vi "Main.vi"(11 "Module Admin":refnum<class "Delacor_lib_QMH_Module Admin.lvclass">) -> ()   [LabVIEW 2025, in "Number Pad.lvlib"]
doc: "This template is based off of the Queued Message Handler design pattern and the Queued Message Handler project template that ships with LabVIEW.\n\nThe main difference is that the queue is private to this module and communication between modules is performed via Broadcast and Request events.\n\nRequest events are wrapped in public API methods and are handled in the Event Handling Loop (EHL) of this VI. Any module can register for Broadcast events sent by this module. The EHL generates messages based on user interface actions.\n\nThe Message Handling Loop (MHL) processes messages generated by the EHL, or by other messages. The messages are string values, so new messages can be added easily to the Message Cases case structure in the MHL. Each message cluster can also provide an optional value for Message Data, which is a variant that can be converted to whatever message-specific data is required.\n_____\nBased on DQMH Dev Tools: Project Template 7.1.0.1503."
uses:
  Number Pad.lvlib
  <vilib>/Delacor/Delacor QMH/Libraries/Module Admin_class/Delacor_lib_QMH_Module Admin.lvclass
  Module Data--cluster.ctl
  <vilib>/Delacor/Delacor QMH/Libraries/Message Queue_class/Delacor_lib_QMH_Message Queue.lvclass/Delacor_lib_QMH_Message Queue.ctl
  Stop Argument--cluster.ctl
  <vilib>/Delacor/Delacor QMH/Libraries/Module Admin_class/Delacor_lib_QMH_Module Admin.lvclass/Delacor_lib_QMH_Module Admin.ctl
  Get VI refnum Argument--cluster.ctl
  Get VI refnum (Reply Payload)--cluster.ctl
  <vilib>/Utility/miscctls.llb/LVPointTypeDef.ctl
  <vilib>/Delacor/Delacor QMH/Libraries/Message Queue_class/Delacor_lib_QMH_Enqueue Message (Single).vi
  <vilib>/Delacor/Delacor QMH/Libraries/Module Admin_class/Delacor_lib_QMH_Get External Launch.vi
  <vilib>/Delacor/Delacor QMH/Libraries/Message Queue_class/Delacor_lib_QMH_Message Queue.lvclass
panel:
  in  "Enter":bool
  out "Buffer Indicator":string
  in  "CLR":bool
  in  "BS":bool
  in  ".":bool
  in  "0":bool
  in  "9":bool
  in  "8":bool
  in  "7":bool
  in  "6":bool
  in  "5":bool
  in  "4":bool
  in  "3":bool
  in  "2":bool
  in  "1":bool
  out "error out":errorcluster
  out "Status":string
  in  "Simulate MHL Error":bool
  in  "Simulate EHL Error":bool
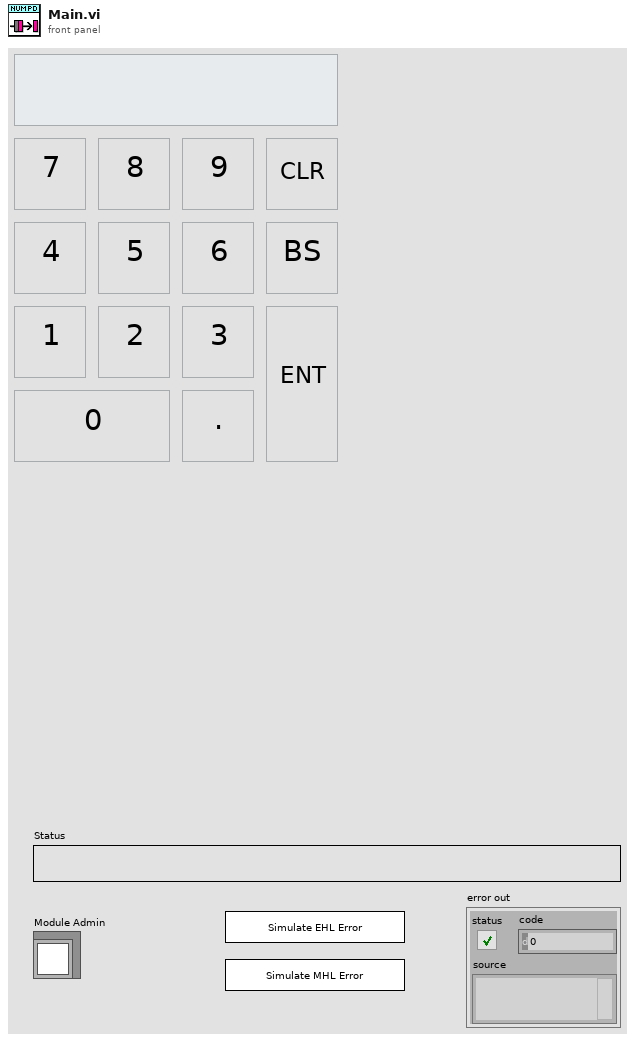
[diagram p1: front panel]
types:
  T1 = typedef "Number Pad.lvlib/Request Events--cluster.ctl" = cluster{"Stop Module":refnum<user-event>, "Show Panel":refnum<user-event>, "Hide Panel":refnum<user-event>, "Get Module Execution Status":refnum<user-event>, "Show Diagram":refnum<user-event>, "Get VI refnum":refnum<user-event>}
  T2 = typedef "Number Pad.lvlib/Module Data--cluster.ctl" = cluster{"Status":string, "Buffer":string}
  T3 = enum32{"invalid lock state", "Not Locked", "Locked (No Password)", "Password-protected"}
  T4 = typedef "Number Pad.lvlib/Stop Argument--cluster.ctl" = cluster{"Origin":string, "Exit via Stop Module Req?":bool, "Wait for Module to stop?":bool}
  T5 = typedef "Number Pad.lvlib/Get VI refnum Argument--cluster.ctl" = cluster{"Wait Notifier":refnum<notifier>, "wait for reply":bool}
  T6 = typedef "LVPointTypeDef.ctl" = cluster{"Horizontal":i16, "Vertical":i16}
  T7 = enum32{"Invalid", "Standard", "Closed", "Hidden", "Minimized", "Maximized"}
  T8 = typedef "Number Pad.lvlib/Get VI refnum (Reply Payload)--cluster.ctl" = cluster{"VI Refnum":refnum<vi>, "error":errorcluster}
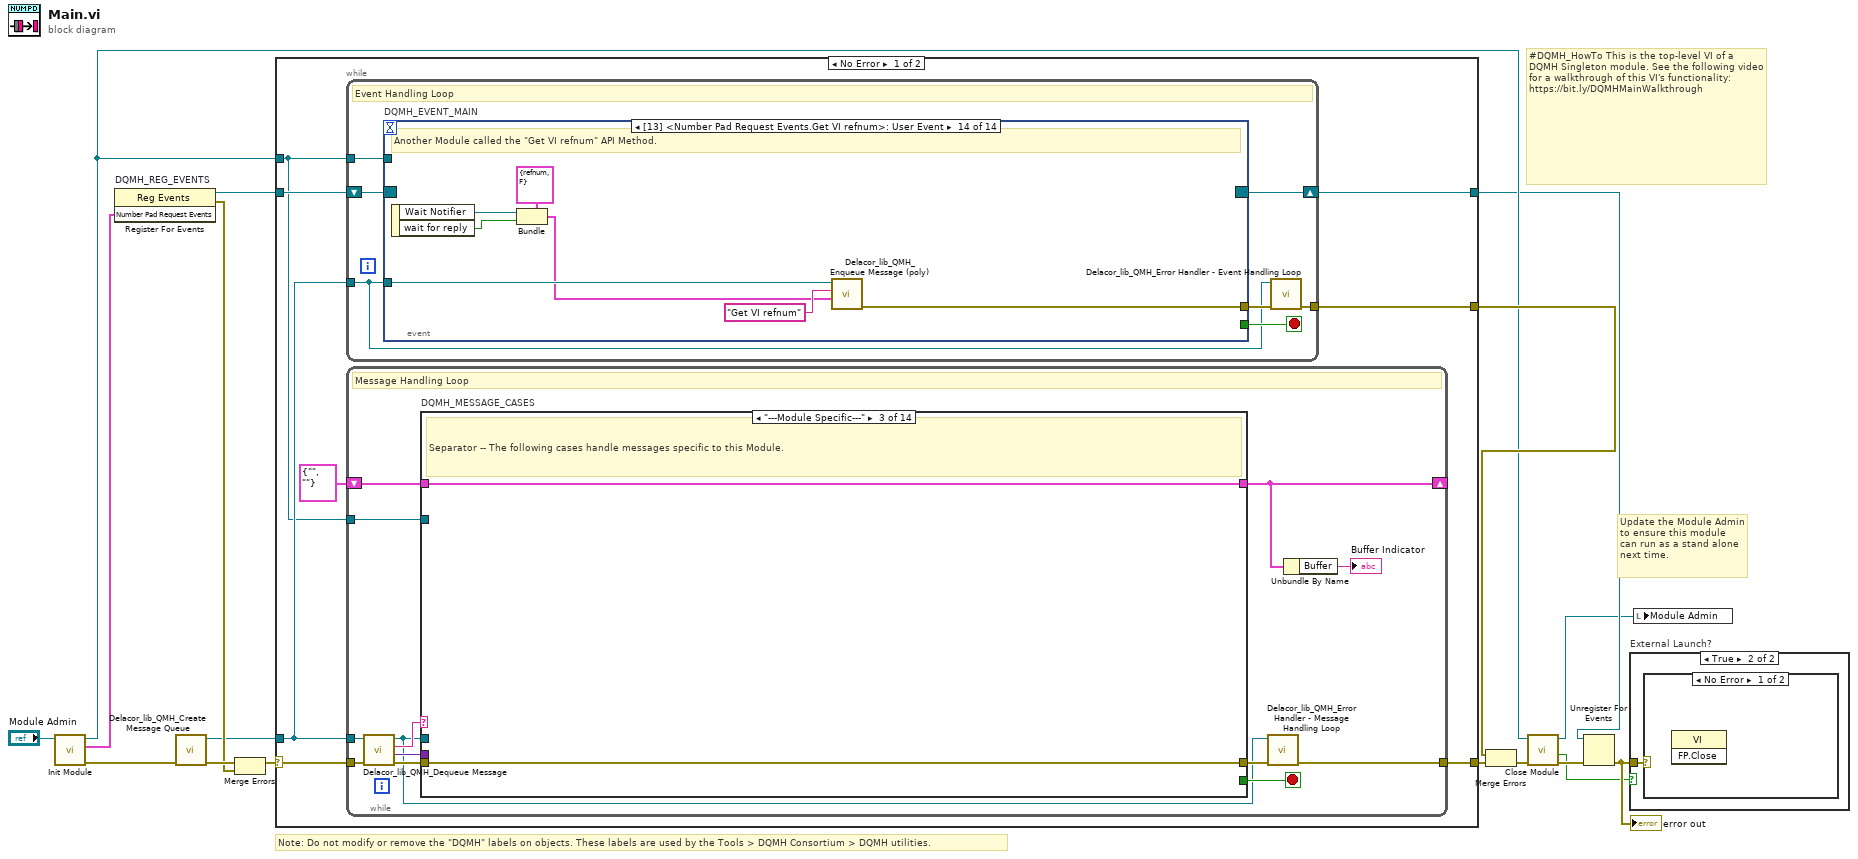
[diagram p0: block diagram]
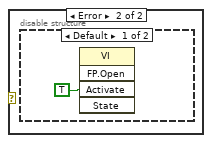
[diagram p3: hidden frame]
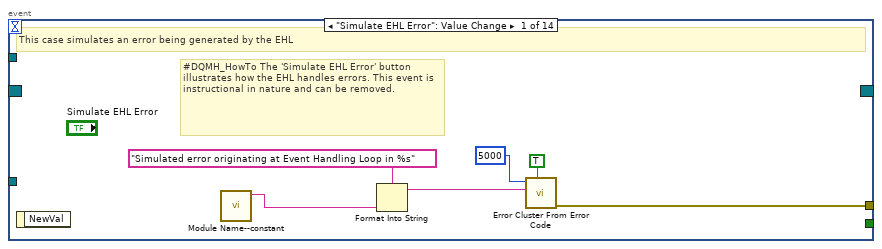
[diagram p5: hidden frame]
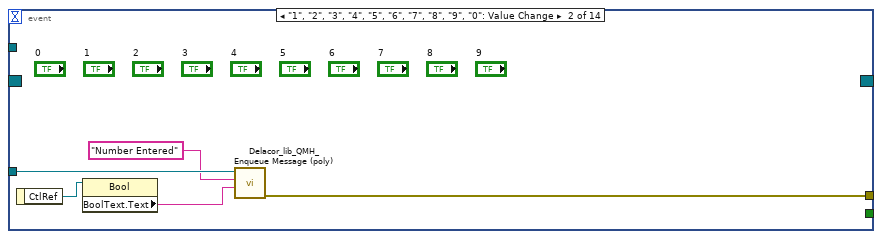
[diagram p6: hidden frame]
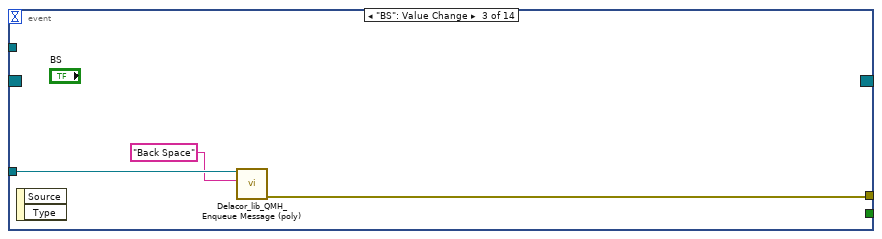
[diagram p7: hidden frame]
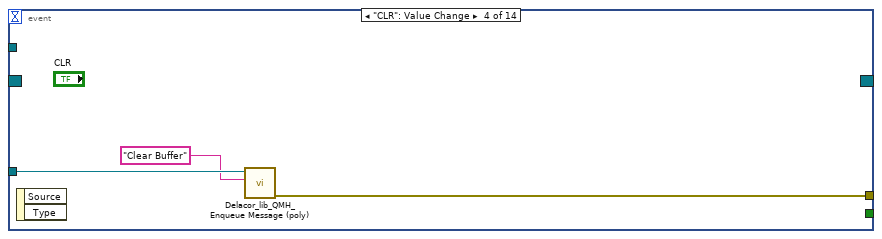
[diagram p8: hidden frame]
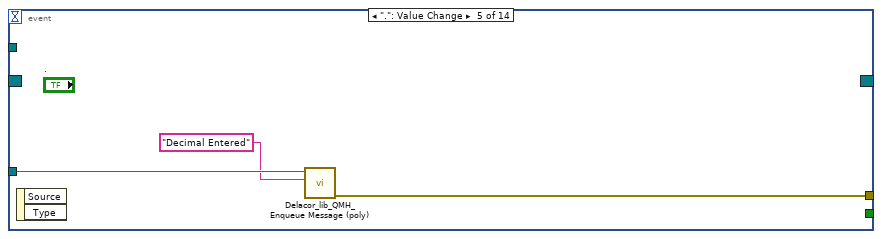
[diagram p9: hidden frame]
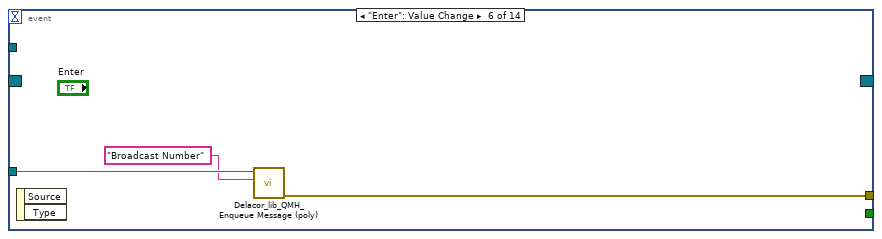
[diagram p10: hidden frame]
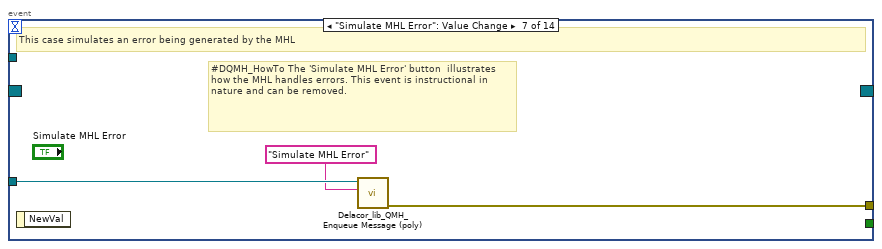
[diagram p11: hidden frame]
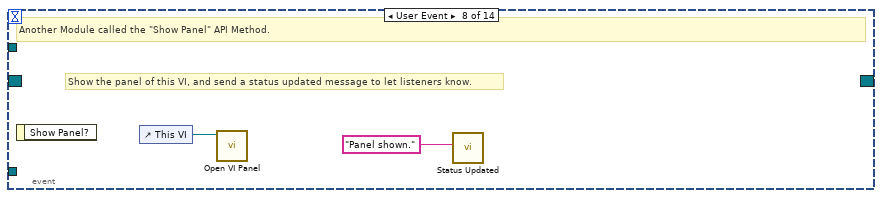
[diagram p12: hidden frame]
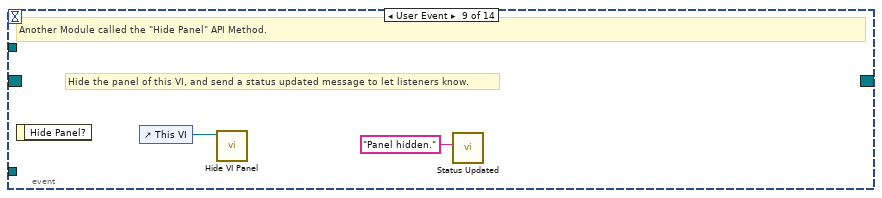
[diagram p13: hidden frame]
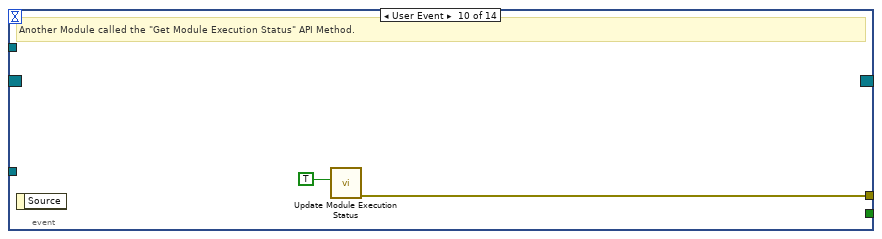
[diagram p14: hidden frame]
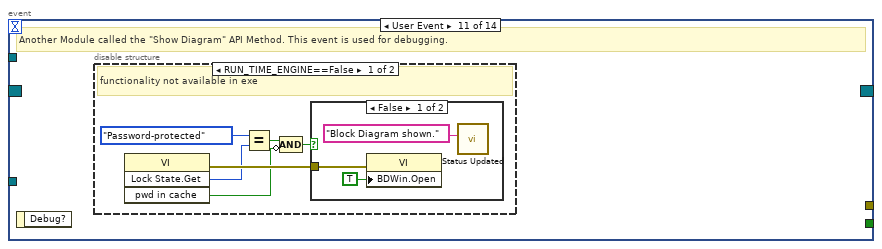
[diagram p15: hidden frame]
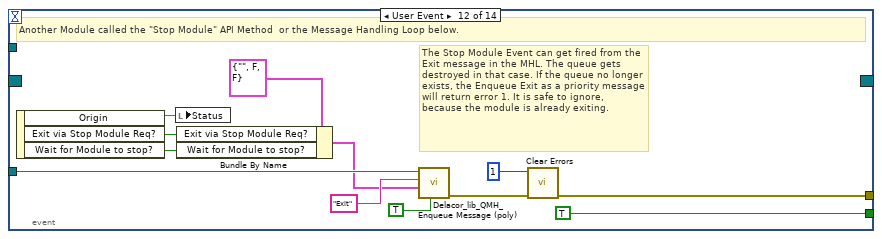
[diagram p18: hidden frame]
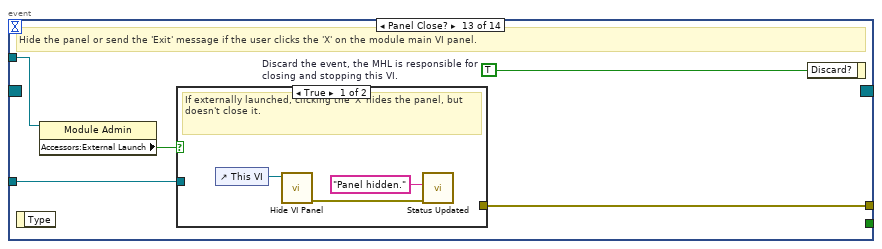
[diagram p19: hidden frame]
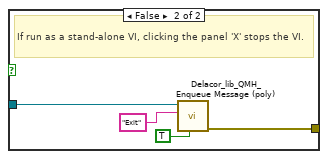
[diagram p20: hidden frame]
diagram:
  # "#DQMH_HowTo This is the top-level VI of a DQMH Singleton module. See the following video for a walkthrough of this VI's functionality: https://bit.ly/DQMHMainWalkthrough"
  # "Note: Do not modify or remove the \"DQMH\" labels on objects. These labels are used by the Tools > DQMH Consortium > DQMH utilities."
  # "Update the Module Admin to ensure this module can run as a stand alone next time."
  n1 = call "Init Module.vi"("Singleton Module Admin in"="Module Admin") -> ("error out"=w16:errorcluster, "Number Pad Request Events"=w5:T1, "Singleton Module Admin out"=w8:refnum<class "Delacor_lib_QMH_Module Admin.lvclass">)  [unwired: 8 in]
  n2 = register-events "DQMH_REG_EVENTS"(w5) -> (reference out=w6:refnum<event-registration>, error out=w9:errorcluster)  [unwired: 2 in]
  n3 = call <vilib>:"Delacor_lib_QMH_Create Message Queue.vi"("error in"=w16) -> ("error out"=w11:errorcluster, "Message Queue"=w4:refnum<class "Delacor_lib_QMH_Message Queue.lvclass">)  [unwired: 9 in]
  n4 = Merge Errors(w11, w9) -> (w10:errorcluster)
  n5 = case shown="No Error" w10 {
    selector: w10 -> [w23 w265]
    tunnel: [w25 w264] -> w17
    tunnel: [w22 w263] -> w7
    tunnel: w6 -> [w20 w263]
    tunnel: w4 -> [w19 w258]
    tunnel: [w24 _] -> w14
    tunnel: w8 -> [w18 w259]
    frame No Error {
      n6 = while {
        tunnel: w19 -> [w26]
        shift-right: [w29] -> w22
        shift-left: w20 -> [w30]
        tunnel: [w31] -> w24
        tunnel: w18 -> [w27]
        stop <- w28 stop-if-true
        # "Event Handling Loop"
        n7 = event "DQMH_EVENT_MAIN" shown="[13] <Number Pad Request Events.Get VI refnum>: User Event" {
          selector: w30 -> [_ _ _ _ _ _ _ _ _ _ _ _ _ _]
          dyn-events: [_ _ _ _ _ _ _ _ _ _ _ _ _ _] -> w29
          timeout: _ -> [_ _ _ _ _ _ _ _ _ _ _ _ _ _]
          tunnel: [_ _ _ _ _ _ _ _ _ _ _ TRUE ("Discard?") _ _] -> w28
          tunnel: w26 -> [_ w43 w46 w49 w52 w55 w57 _ _ _ _ w81 w88 w104]
          tunnel: [w38 w42 w45 w48 w51 w54 w58 _ _ w64 _ w84 w90 w98] -> w32
          tunnel: w27 -> [_ _ _ _ _ _ _ _ _ _ _ _ w87 _]
          event "Simulate EHL Error": Value Change {
            # "#DQMH_HowTo The 'Simulate EHL Error' button  illustrates how the EHL handles errors. This event is instructional in nature and can be removed."
            # "This case simulates an error being generated by the EHL"
            n8 = event-data() -> ()  [unwired: 1 in, 1 out]
            n9 = call "Module Name--constant.vi"() -> ("Module Name"=w35:string)  [unwired: 11 in]
            n10 = Format Into String(format string="Simulated error originating at Event Handling Loop in %s", w35) -> (resulting string=w36:string)  [unwired: 2 in, 1 out]
            n11 = call <vilib>:"Error Cluster From Error Code.vi"("show call chain? (False)"=TRUE, "error message (\"\")"=w36, "error code (0)"=5000) -> ("error out"=w38:errorcluster)  [unwired: 6 in]
          }
          event "1", "2", "3", "4", "5", "6", "7", "8", "9", "0": Value Change {
            n12 = event-data() -> ("CtlRef"=w40:refnum<vi>)  [unwired: 1 in]
            n13 = property class="Bool"(reference=w40) -> ("BoolText.Text"=w39:string)  [unwired: 1 in, 2 out]
            n14 = call-poly <vilib>:"Delacor_lib_QMH_Enqueue Message (poly).vi"("Message Data"=w39, "Message"="Number Entered", "Message Queue in"=w43) -> ("error out"=w42:errorcluster)  [unwired: 7 in, 1 out]
          }
          event "BS": Value Change {
            n15 = event-data() -> ()  [unwired: 1 in, 2 out]
            n16 = call-poly <vilib>:"Delacor_lib_QMH_Enqueue Message (poly).vi"("Message"="Back Space", "Message Queue in"=w46) -> ("error out"=w45:errorcluster)  [unwired: 8 in, 1 out]
          }
          event "CLR": Value Change {
            n17 = event-data() -> ()  [unwired: 1 in, 2 out]
            n18 = call-poly <vilib>:"Delacor_lib_QMH_Enqueue Message (poly).vi"("Message"="Clear Buffer", "Message Queue in"=w49) -> ("error out"=w48:errorcluster)  [unwired: 8 in, 1 out]
          }
          event ".": Value Change {
            n19 = event-data() -> ()  [unwired: 1 in, 2 out]
            n20 = call-poly <vilib>:"Delacor_lib_QMH_Enqueue Message (poly).vi"("Message"="Decimal Entered", "Message Queue in"=w52) -> ("error out"=w51:errorcluster)  [unwired: 8 in, 1 out]
          }
          event "Enter": Value Change {
            n21 = event-data() -> ()  [unwired: 1 in, 2 out]
            n22 = call-poly <vilib>:"Delacor_lib_QMH_Enqueue Message (poly).vi"("Message"="Broadcast Number", "Message Queue in"=w55) -> ("error out"=w54:errorcluster)  [unwired: 8 in, 1 out]
          }
          event "Simulate MHL Error": Value Change {
            # "#DQMH_HowTo The 'Simulate MHL Error' button  illustrates how the MHL handles errors. This event is instructional in nature and can be removed."
            # "This case simulates an error being generated by the MHL"
            n23 = event-data() -> ()  [unwired: 1 in, 1 out]
            n24 = call-poly <vilib>:"Delacor_lib_QMH_Enqueue Message (poly).vi"("Message"="Simulate MHL Error", "Message Queue in"=w57) -> ("error out"=w58:errorcluster)  [unwired: 8 in, 1 out]
          }
          event User Event {
            # "Show the panel of this VI, and send a status updated message to let listeners know."
            # "Another Module called the \"Show Panel\" API Method."
            n25 = event-data() -> ()  [unwired: 1 in, 1 out]
            n26 = control-ref of="This VI"() -> (w60:refnum<vi>)
            n27 = call "Open VI Panel.vi"("VI"=w60) -> ()  [unwired: 10 in, 1 out]
            n28 = call "Status Updated.vi"("Status"="Panel shown." ("format string")) -> ()  [unwired: 10 in, 1 out]
          }
          event User Event {
            # "Hide the panel of this VI, and send a status updated message to let listeners know."
            # "Another Module called the \"Hide Panel\" API Method."
            n29 = event-data() -> ()  [unwired: 1 in, 1 out]
            n30 = control-ref of="This VI"() -> (w62:refnum<vi>)
            n31 = call "Hide VI Panel.vi"("VI"=w62) -> ()  [unwired: 10 in, 1 out]
            n32 = call "Status Updated.vi"("Status"="Panel hidden." ("format string")) -> ()  [unwired: 10 in, 1 out]
          }
          event User Event {
            # "Another Module called the \"Get Module Execution Status\" API Method."
            n33 = event-data() -> ()  [unwired: 1 in, 1 out]
            n34 = call "Update Module Execution Status.vi"("Running?"=TRUE) -> ("error out"=w64:errorcluster)  [unwired: 10 in]
          }
          event User Event {
            # "Another Module called the \"Show Diagram\" API Method. This event is used for debugging."
            n35 = event-data() -> ()  [unwired: 1 in, 1 out]
            n36 = disable-structure shown="RUN_TIME_ENGINE==False" {
              frame condition #0 (active) {
                # "functionality not available in exe"
                n37 = invoke on="Invoke Node" class="VI" method="Lock State.Get"() -> (error out=w70:errorcluster, "Get Lock State"=w69:T3, "pwd in cache"=w66:bool)  [unwired: 4 in, 1 out]
                n38 = Equal?(x=T3."Password-protected", y=w69) -> (x = y?=w67:bool)
                n39 = Compound Arithmetic op=AND(w67, invert w66) -> (w65:bool)
                n40 = case shown="False" w65 {
                  tunnel: w70 -> [w73 _]
                  frame False {
                    n41 = property on="Property Node" class="VI"(error in=w73, "BDWin.Open"=TRUE ("Block Diagram Window:Open")) -> ()  [unwired: 1 in, 2 out]
                    n42 = call "Status Updated.vi"("Status"="Block Diagram shown." ("format string")) -> ()  [unwired: 10 in, 1 out]
                  }
                  frame True {
                    # "Password-protected VI, and the password is not in the cache. Do not show the diagram."
                  }
                }
              }
              frame condition #1 {
              }
            }
          }
          event User Event {
            # "The Stop Module Event can get fired from the Exit message in the MHL. The queue gets destroyed in that case. If the queue no longer exists, the Enqueue Exit as a priority message will return error 1. It is safe to ignore, because the module is already exiting."
            # "Another Module called the \"Stop Module\" API Method  or the Message Handling Loop below."
            n43 = event-data() -> ("Origin"=w80:string, "Exit via Stop Module Req?"=w76:bool, "Wait for Module to stop?"=w75:bool)  [unwired: 1 in]
            n44 = local write "Status"(w80) -> ()
            n45 = Bundle By Name(cluster=T4 {"Origin"="", "Exit via Stop Module Req?"=FALSE, "Wait for Module to stop?"=FALSE} ("Stop Argument"), "Exit via Stop Module Req?"=w76, "Wait for Module to stop?"=w75) -> (w74:T4)
            n46 = call-poly <vilib>:"Delacor_lib_QMH_Enqueue Message (poly).vi"("Priority Message? (F)"=TRUE, "Message Data"=w74, "Message"="Exit", "Message Queue in"=w81) -> ("error out"=w85:errorcluster)  [unwired: 6 in, 1 out]
            n47 = call <vilib>:"Clear Errors.vi"("error in (no error)"=w85, "specific error code to clear (0: all)"=1) -> ("error out"=w84:errorcluster)  [unwired: 4 in, 1 out]
          }
          event Panel Close? {
            w89 = TRUE  # Discard the event, the MHL is responsible for closing and stopping this VI.
            # "Hide the panel or send the 'Exit' message if the user clicks the 'X' on the module main VI panel."
            n48 = event-data() -> ()  [unwired: 1 in, 1 out]
            n49 = property on="Property Node" class="Module Admin"(reference=w87) -> ("Accessors:External Launch"=w86:bool)  [unwired: 1 in, 2 out]
            n50 = case shown="True" w86 {
              tunnel: w88 -> [_ w96]
              tunnel: [_ w97] -> w90
              frame True {
                # "If externally launched, clicking the 'X' hides the panel, but doesn't close it."
                n51 = control-ref of="This VI"() -> (w93:refnum<vi>)
                n52 = call "Hide VI Panel.vi"("VI"=w93) -> ("error out"=w91:errorcluster)  [unwired: 10 in]
                n53 = call "Status Updated.vi"("error in"=w91, "Status"="Panel hidden." ("format string")) -> ()  [unwired: 9 in, 1 out]
              }
              frame False {
                # "If run as a stand-alone VI, clicking the panel 'X' stops the VI."
                n54 = call-poly <vilib>:"Delacor_lib_QMH_Enqueue Message (poly).vi"("Priority Message? (F)"=TRUE, "Message"="Exit", "Message Queue in"=w96) -> ("error out"=w97:errorcluster)  [unwired: 7 in, 1 out]
              }
            }
            n55 = event-data ("Event Filter Node")("Discard?"=w89) -> ()  [unwired: 1 in, 1 out]
          }
          event User Event {
            # "Another Module called the \"Get VI refnum\" API Method."
            n56 = event-data() -> ("Wait Notifier"=w100:refnum<notifier>, "wait for reply"=w99:bool)  [unwired: 1 in]
            n57 = Bundle(cluster=T5 {"Wait Notifier"=refnum, "wait for reply"=FALSE} ("Get VI refnum Argument"), "Wait Notifier"=w100, "wait for reply"=w99) -> (w101:T5)
            n58 = call-poly <vilib>:"Delacor_lib_QMH_Enqueue Message (poly).vi"("Message Data"=w101, "Message"="Get VI refnum", "Message Queue in"=w104) -> ("error out"=w98:errorcluster)  [unwired: 7 in, 1 out]
          }
        }
        n59 = call-dynamic "Delacor_lib_QMH_Error Handler - Event Handling Loop.vi"("error in"=w32, "Message Queue in"=w26) -> ("dup error in"=w31:errorcluster)  [unwired: 8 in, 1 out]
      }
      n60 = while {
        tunnel: w19 -> [w107]
        shift-right: [w106] -> _
        shift-left: T2 {"Status"="", "Buffer"=""} ("Data Cluster") -> [w115]
        tunnel: w23 -> [w117]
        tunnel: [w110] -> w25
        tunnel: w18 -> [w111]
        stop <- w114 stop-if-true
        # "Message Handling Loop"
        n61 = call-dynamic "Delacor_lib_QMH_Dequeue Message.vi"("error in"=w117, "Message Queue in"=w107) -> ("error out"=w116:errorcluster, "Message Data"=w112:variant, "Message"=w113:string, "Message Queue out"=w108:refnum<class "Delacor_lib_QMH_Message Queue.lvclass">)  [unwired: 6 in]
        n62 = case "DQMH_MESSAGE_CASES" shown="\"---Module Specific---\"" w113 {
          selector: w113 -> [_ _ _ _ _ _ _ _ _ _ _ _ _ w253]
          tunnel: w108 -> [_ _ _ _ _ _ _ _ _ _ _ w219 w241 _]
          tunnel: w116 -> [w135 w140 w142 w149 w159 w173 w181 w193 w197 w206 w215 w226 w247 w256]
          tunnel: [w133 w139 w142 w148 w159 w173 w181 w183 w196 w206 w214 w222 w242 w257] -> w109
          tunnel: w115 -> [w124 w138 w141 w145 w158 w172 w180 w192 w199 w205 w212 w221 w240 w254]
          tunnel: [w123 w138 w141 w143 w154 w171 w179 w192 w199 w205 w212 w221 w240 w254] -> w106
          tunnel: [_ _ _ _ _ _ _ _ _ _ _ _ w239 _] -> w114
          tunnel: w112 -> [_ _ _ w147 _ _ _ w190 _ _ _ w220 w238 _]
          tunnel: w111 -> [w125 _ _ _ _ _ _ _ _ _ _ w218 w233 _]
          frame "Initialize" {
            w119 = "Initial Message" ("Initial Message")
            # "#DQMH_CodeNeeded - Initialize the appearance of the front panel."
            # "#DQMH_CodeNeeded - Initialize your state data here."
            # "Initialize - Any operation that needs to be done before the module can receive messages. Synchronize Caller Events.vi will inform Start Module.vi that the module has launched and is ready to receive messages. Module Did Init.vi will broadcast that the module initialized."
            n63 = call "Synchronize Caller Events.vi"("error in"=w135, "Singleton Module Admin in"=w125) -> ("error out"=w134:errorcluster, "Singleton Module Admin out"=w120:refnum<class "Delacor_lib_QMH_Module Admin.lvclass">)  [unwired: 8 in]
            n64 = property on="Property Node" class="Module Admin"(reference=w120) -> ("Accessors:External Launch"=w129:bool)  [unwired: 1 in, 2 out]
            n65 = Select(t=T7."Hidden" ("State"), s=w129, f=T7."Standard" ("State")) -> (s? t:f=w126:T7)
            n66 = call "Module Name--constant.vi"() -> ("Module Name"=w132:string)  [unwired: 11 in]
            n67 = property on="Property Node" class="VI"("Front Panel.Title"=w132) -> (reference out=w131:refnum<vi>, error out=w137:errorcluster)  [unwired: 2 in]
            n68 = invoke on="Invoke Node" class="VI" method="FP.Open"(reference=w131, error in=w137, "State"=w126) -> (reference out=w130:refnum<vi>, error out=w136:errorcluster)  [unwired: 2 in, 3 out]
            n69 = Bundle By Name(cluster=w124, "Status"=w119) -> (w123:T2)
            n70 = invoke on="Invoke Node" class="VI" method="FP.Center"(reference=w130, error in=w136) -> ()  [unwired: 1 in, 3 out]
            n71 = property on="Pane" class="Pane"("Origin"=T6 {"Horizontal"=0, "Vertical"=0}) -> ()  [unwired: 2 in, 2 out]
            n72 = call "Module Name--constant.vi"() -> ("Module Name"=w121:string)  [unwired: 11 in]
            n73 = call "Module Did Init.vi"("error in"=w134, "Initialized?"=TRUE, "Origin"=w121) -> ("error out"=w133:errorcluster)  [unwired: 8 in]
            "Status" <- w119
          }
          frame "---Copy This Frame---" {
            # "Duplicate this frame when creating new messages.  Change this comment in the duplicated frame to describe this message."
            n74 = Merge Errors(w140) -> (w139:errorcluster)
          }
          frame "---Module Specific---" {
            # "Separator -- The following cases handle messages specific to this Module."
          }
          frame "Number Entered" {
            # "Update buffer"
            n75 = Variant To Data(error in=w149, type="", Variant=w147) -> (data=w144:string, error out=w148:errorcluster)
            n76 = in-place {
              in-place-border: w144 -> [w151]
              n77 = in-place-cluster #1(w145) -> ("Buffer"=w152:string)
              n78 = Concatenate Strings(w152, w151) -> (w150:string)
              n79 = in-place-cluster #1("Buffer"=w150) -> (w143:T2)
            }
          }
          frame "Decimal Entered" {
            n80 = Unbundle By Name(w158) -> ("Buffer"=w155:string)
            n81 = Equal?(x=w155, y="") -> (x = y?=w156:bool)
            n82 = case shown="False" w156 {
              tunnel: [w160 "0."] -> w153
              tunnel: w155 -> [w161 _]
              frame False {
                # "Buffer not empty.\nCheck for an existing decimal."
                n83 = Match Pattern(string=w161, regular expression="[.]") -> (match substring=w164:string)  [unwired: 1 in, 3 out]
                n84 = Equal?(x=w164, y=".") -> (x = y?=w162:bool)
                n85 = case shown="True" w162 {
                  tunnel: w161 -> [w168 w169]
                  tunnel: [w167 w169] -> w160
                  frame False {
                    # "No decimal.\nAdd one."
                    n86 = Concatenate Strings(w168, "." ("string")) -> (w167:string)
                  }
                  frame True {
                    # "Decimal exists.\nDon't add one."
                  }
                }
              }
              frame True {
                # "Buffer is empty. Add a zero and a decimal."
              }
            }
            n87 = Bundle By Name(cluster=w158, "Buffer"=w153) -> (w154:T2)
          }
          frame "Back Space" {
            # "Convert to byte array give a quick array\nto work with. Remove the last entered \nelement (by default - hence no need to\nspecify lenght or index)."
            n88 = in-place {
              n89 = in-place-cluster #2(w172) -> ("Buffer"=w177:string)
              n90 = String To Byte Array(string=w177) -> (unsigned byte array=w176:u8[])
              n91 = Delete From Array(array=w176) -> (array with subset deleted=w175:u8[])  [unwired: 2 in, 1 out]
              n92 = Byte Array To String(unsigned byte array=w175) -> (string=w174:string)
              n93 = in-place-cluster #2("Buffer"=w174) -> (w171:T2)
            }
          }
          frame "Clear Buffer" {
            # "Clear out the buffer."
            n94 = Bundle By Name(cluster=w180, "Buffer"="") -> (w179:T2)
          }
          frame "Get VI refnum" {
            # "Retrive the VI refnum. This is typically used for inserting this module into a subpanel."
            n95 = Variant To Data(error in=w193, type=T5 {"Wait Notifier"=refnum, "wait for reply"=FALSE} ("Get VI refnum Argument"), Variant=w190) -> (data=w188:T5, error out=w191:errorcluster)
            n96 = Unbundle By Name(w188) -> ("Wait Notifier"=w187:refnum<notifier>, "wait for reply"=w186:bool)
            n97 = control-ref of="This VI"() -> (w182:refnum<vi>)
            n98 = Bundle By Name(cluster=T8 {"VI Refnum"=refnum, "error"={"status"=FALSE, "code"=0, "source"=""}} ("Get VI refnum (Reply Payload)"), "VI Refnum"=w182) -> (w185:T8)
            n99 = Merge Errors(w191) -> (w183:errorcluster)
            n100 = case "DQMH_FIRE_NOTIFIER" shown="True" w186 {
              tunnel: w187 -> [_ w195]
              tunnel: w185 -> [_ w194]
              frame False {
              }
              frame True {
                n101 = Send Notification(notification=w194, notifier=w195) -> ()  [unwired: 1 in, 2 out]
              }
            }
          }
          frame "Broadcast Number" {
            # "Don't send a zero and a decimal. When would that beneeded?\n\nAlthough, allow an empty string to be sent. That could be use to clear out a field."
            n102 = Unbundle By Name(w199) -> ("Buffer"=w198:string)
            n103 = case shown="Default" w198 {
              selector: w198 -> [w202 _]
              tunnel: w197 -> [w201 w204]
              tunnel: [w200 w204] -> w196
              frame Default {
                n104 = Fract/Exp String To Number(string=w202) -> (number=w203:dbl)  [unwired: 3 in, 1 out]
                n105 = call "Send Number.vi"("error in"=w201, "Number Numeric"=w203, "Number String"=w202) -> ("error out"=w200:errorcluster)  [unwired: 8 in]
              }
              frame "0." {
              }
            }
          }
          frame "---Exit and Error Handling---" {
            # "Separator - The following cases handle errors and exit messages."
          }
          frame "Simulate MHL Error" {
            # "#DQMH_HowTo The 'Simulate MHL Error' button  illustrates how the MHL handles errors. This event is instructional in nature and can be removed."
            # "Simulate an error occurring at the MHL"
            n106 = call "Module Name--constant.vi"() -> ("Module Name"=w208:string)  [unwired: 11 in]
            n107 = Format Into String(format string="Simulated error originating at Message Handling Loop in %s", w208) -> (resulting string=w209:string)  [unwired: 2 in, 1 out]
            n108 = call <vilib>:"Error Cluster From Error Code.vi"("show call chain? (False)"=TRUE, "error message (\"\")"=w209, "error code (0)"=5001) -> ("error out"=w213:errorcluster)  [unwired: 6 in]
            n109 = Merge Errors(w215, w213) -> (w214:errorcluster)
          }
          frame "Error" {
            # "#DQMH_CodeRecommended - If the module is running in standalone mode (External Launch = FALSE), this code will pop up an error dialog and call the 'Exit' message if an error occurs. Add more fine-grained error management here."
            # "Error - Check the error message data and respond accordingly. This message is sent by the \"Error Handler\" VIs at the end of each loop in this application."
            n110 = property on="Property Node" class="Module Admin"(reference=w218) -> ("Accessors:External Launch"=w217:bool)  [unwired: 1 in, 2 out]
            n111 = Variant To Data(error in=w226, type=errorcluster {"status"=FALSE, "code"=0, "source"=""} ("error constant"), Variant=w220) -> (data=w216:errorcluster, error out=w224:errorcluster)
            n112 = local write "error out"(w216) -> ()
            n113 = call "Error Reported.vi"("Error"=w216) -> ()  [unwired: 10 in, 1 out]
            n114 = case shown="False" w217 {
              tunnel: [w231 _] -> w223
              tunnel: w219 -> [w229 _]
              tunnel: w216 -> [w230 _]
              frame False {
                n115 = disable-structure shown="Default" {
                  disable-tunnel: w230 -> [w232 _]
                  frame condition #0 (active) {
                    # "If the module is running standalone, then pop up an error dialog and call the \"Exit\" message."
                    n116 = call <vilib>:"Simple Error Handler.vi"("error in (no error)"=w232) -> ()  [unwired: 4 in, 5 out]
                  }
                  frame condition #1 {
                    # "To prevent the Simple Error Handler VI from being loaded (e.g. when deploying to a Real-Time target), add the Conditional Disable Symbol \"DQMH_Disable_SEH\" to your project and set it to TRUE."
                  }
                }
                n117 = call-poly <vilib>:"Delacor_lib_QMH_Enqueue Message (poly).vi"("Priority Message? (F)"=TRUE, "Message"="Exit", "Message Queue in"=w229) -> ("error out"=w231:errorcluster)  [unwired: 7 in, 1 out]
              }
              frame True {
                # "If the module was launched externally, calling the Error Reported broadcast VI is the only action performed by the \"Error\" message. The module's caller can then process the error appropriately."
              }
            }
            n118 = Merge Errors(w224, w223) -> (w222:errorcluster)
          }
          frame "Exit" {
            w237 = 91  # 91: not all Exit messages will have an argument
            w239 = TRUE  # Stop the VI
            # "Release the message queue reference"
            # "#DQMH_CodeNeeded - Add any required cleanup code here."
            # "Exit - Exit the application."
            n119 = Variant To Data(error in=w247, type=T4 {"Origin"="", "Exit via Stop Module Req?"=FALSE, "Wait for Module to stop?"=FALSE} ("Stop Argument"), Variant=w238) -> (data=w235:T4, error out=w244:errorcluster)
            n120 = call <vilib>:"Clear Errors.vi"("error in (no error)"=w244, "specific error code to clear (0: all)"=w237) -> ("error out"=w246:errorcluster)  [unwired: 4 in, 1 out]
            n121 = control-ref of="This VI"() -> (w234:refnum<vi>)
            n122 = call-dynamic "Delacor_lib_QMH_Release Message Queue.vi"("error in"=w246, "Message Queue"=w241) -> ("error out"=w245:errorcluster)  [unwired: 9 in]
            n123 = call "Handle Exit.vi"("Stop Argument"=w235, "Admin in"=w233, "VI reference"=w234) -> ("error out"=w243:errorcluster)  [unwired: 7 in, 1 out]
            n124 = Merge Errors(w245, w243) -> (w242:errorcluster)
            n125 = call "Error Reported.vi"("Error"=w242) -> ()  [unwired: 10 in, 1 out]
          }
          frame Default {
            # "'Default' case only runs if there is a message that isn't defined in any of the other cases.  Output a programming error."
            n126 = call "Module Name--constant.vi"() -> ("Module Name"=w252:string)  [unwired: 11 in]
            n127 = Format Into String(format string="The invalid message string \"%s\" was received in the Message Handling Loop for module \"%s\".", w253, w252) -> (resulting string=w248:string)  [unwired: 2 in, 1 out]
            n128 = call <vilib>:"Error Cluster From Error Code.vi"("show call chain? (False)"=TRUE, "error message (\"\")"=w248, "error code (0)"=1) -> ("error out"=w255:errorcluster)  [unwired: 6 in]
            n129 = Merge Errors(w256, w255) -> (w257:errorcluster)
          }
        }
        n130 = call-dynamic "Delacor_lib_QMH_Error Handler - Message Handling Loop.vi"("error in"=w109, "Message Queue in"=w108) -> ("dup error in"=w110:errorcluster)  [unwired: 8 in, 1 out]
        n131 = Unbundle By Name(w106) -> ("Buffer"=→"Buffer Indicator":string)
      }
    }
    frame Error {
      # "Synchronize Caller Events.vi will inform Start Module.vi that the module has launched and will let the code calling Start Module.vi register for broadcasts and would permit the caller receive the broadcast that an error occurred at launch time."
      n132 = call-dynamic "Delacor_lib_QMH_Release Message Queue.vi"("error in"=w265, "Message Queue"=w258) -> ("error out"=w264:errorcluster)  [unwired: 9 in]
      n133 = call "Synchronize Caller Events.vi"("Singleton Module Admin in"=w259) -> ("error out"=w266:errorcluster)  [unwired: 9 in, 1 out]
      n134 = call "Module Name--constant.vi"() -> ("Module Name"=w262:string)  [unwired: 11 in]
      n135 = Format Into String(format string="An error occurred during initialization. %s is no longer running.", w262) -> (resulting string=w260:string)  [unwired: 2 in, 1 out]
      n136 = Merge Errors(w264, w266) -> (w267:errorcluster)
      n137 = call "Error Reported.vi"("Additional Information"=w260, "Error"=w267) -> ()  [unwired: 9 in, 1 out]
    }
  }
  n138 = Merge Errors(w14, w17) -> (w13:errorcluster)
  n139 = call "Close Module.vi"("error in"=w13, "Module Admin in"=w8) -> ("error out"=w15:errorcluster, "External Launch"=w1:bool, "Module Admin out"=w2:refnum<class "Delacor_lib_QMH_Module Admin.lvclass">)  [unwired: 7 in]
  n140 = Unregister For Events(event registration refnum=w7, error in=w15) -> (error out=w12:errorcluster)
  "error out" <- w12
  n141 = case "External Launch?" shown="True" w1 {
    tunnel: w12 -> [_ w268]
    frame False {
    }
    frame True {
      n142 = case shown="No Error" w268 {
        frame No Error {
          n143 = invoke on="Invoke Node" class="VI" method="FP.Close"() -> ()  [unwired: 3 in, 3 out]
        }
        frame Error {
          n144 = disable-structure shown="Default" {
            frame condition #0 (active) {
              n145 = invoke class="VI" method="FP.Open"("Activate"=TRUE ("Activate?")) -> ()  [unwired: 4 in, 5 out]
            }
            frame condition #1 {
              # "Don't show panel on error if running inside a built EXE."
            }
          }
        }
      }
    }
  }
  n146 = local write "Module Admin"(w2) -> ()
